vi "GetCellTypesAndValues.vi"(11 "XML":string) -> (2 "Type":string[](array[string]), 3 "Value":string[](array[string]))   [LabVIEW 2013]
uses:
  XML.lvlib
  <vilib>/xml/NI_XML.lvlib
  <resource>/objmgr/DOMUserDefRef.rc
panel:
  # "Output"
  # "Input"
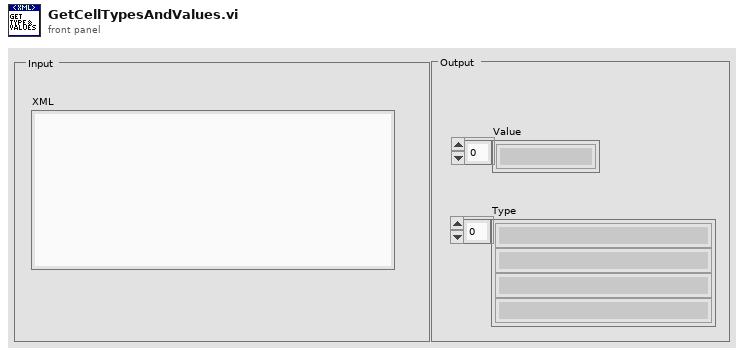
[diagram p1: front panel]
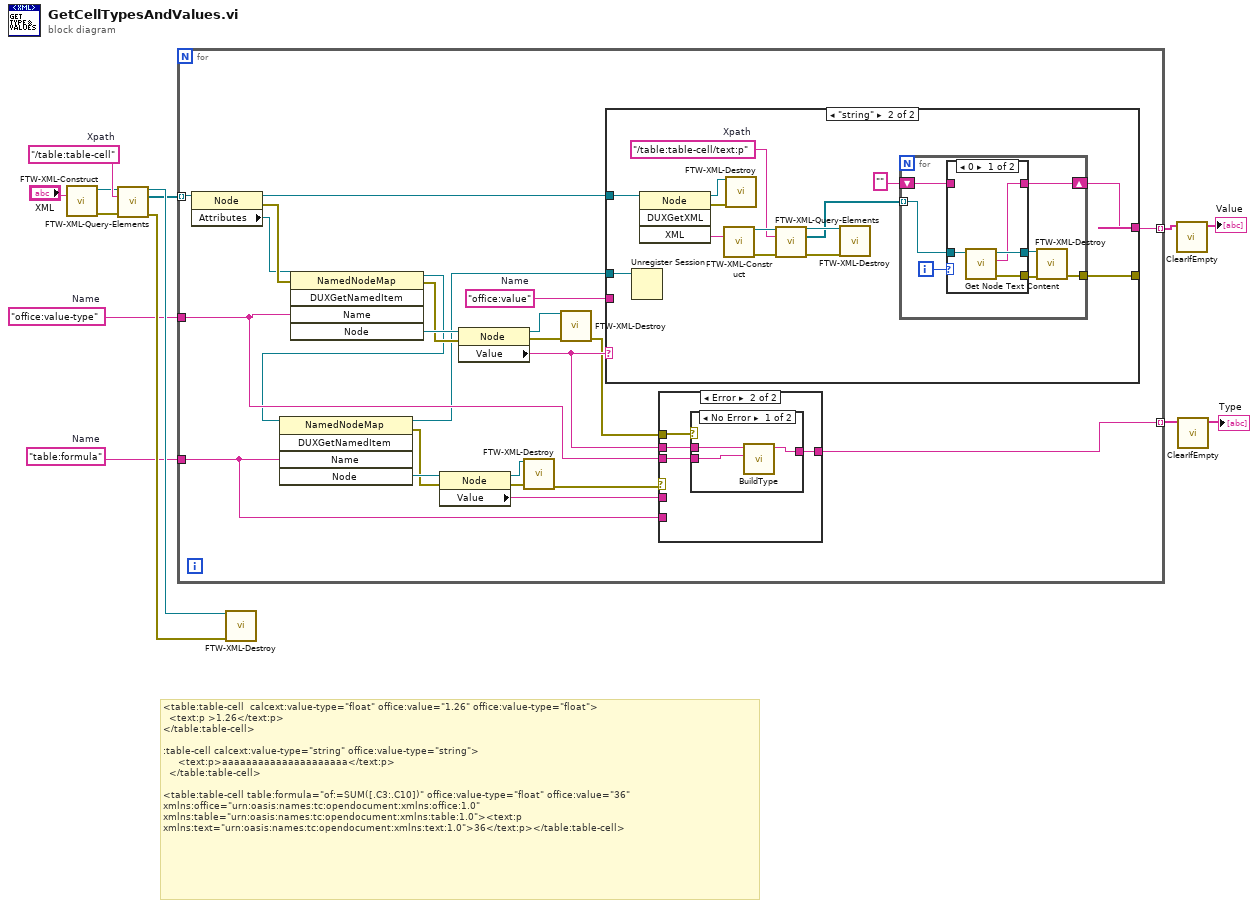
[diagram p0: block diagram]
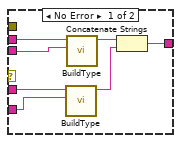
[diagram p2: hidden frame]
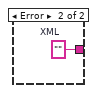
[diagram p3: hidden frame]
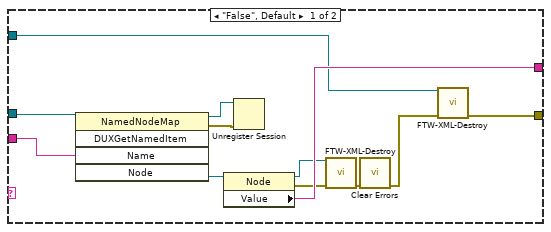
[diagram p4: hidden frame]
diagram:
  w5 = "table:formula"  # Name
  w6 = "office:value-type"  # Name
  w10 = "/table:table-cell"  # Xpath
  # "<table:table-cell  calcext:value-type=\"float\" office:value=\"1.26\" office:value-type=\"float\">\n  <text:p >1.26</text:p>\n</table:table-cell>\n\n:table-cell calcext:value-type=\"string\" office:value-type=\"string\">           \n     <text:p>aaaaaaaaaaaaaaaaaaaaa</text:p>\n  </table:table-cell>\n\n<table:table-cell table:formula=\"of:=SUM([.C3:.C10])\" office:value-type=\"float\" office:value=\"36\" xmlns:office=\"urn:oasis:names:tc:opendocument:xmlns:office:1.0\" xmlns:table=\"urn:oasis:names:tc:opendocument:xmlns:table:1.0\"><text:p xmlns:text=\"urn:oasis:names:tc:opendocument:xmlns:text:1.0\">36</text:p></table:table-cell>"
  n1 = call "FTW-XML-Construct.vi"("XML String"="XML") -> ("XML Document"=w8:refnum<k20>, "error out"=w9:errorcluster)  [unwired: 13 in]
  n2 = call "FTW-XML-Query-Elements.vi"("XML Node"=w8, "XPath Query"=w10, "error in"=w9) -> ("XML Node out"=w13:refnum<k20>, "Matching Nodes"=w11:refnum<k20>[], "error out"=w12:errorcluster)  [unwired: 9 in, 1 out]
  n3 = for {
    tunnel: [w36] -> w4 mode=indexing
    tunnel: w11 -> [w35] mode=indexing
    tunnel: w6 -> [w20]
    tunnel: [w23] -> w2 mode=indexing
    tunnel: w5 -> [w21]
    w29 = "office:value"  # Name
    n4 = property class="Node"(reference=w35) -> (reference out=w28:refnum<k20>, error out=w34:errorcluster, "Attributes"=w27:refnum<k20>)  [unwired: 1 in]
    n5 = invoke class="NamedNodeMap" method="DUXGetNamedItem"(reference=w27, error in=w34, "Name"=w20) -> (reference out=w15:refnum<k20>, error out=w30:errorcluster, "Node"=w33:refnum<k20>)  [unwired: 2 in, 2 out]
    n6 = invoke class="NamedNodeMap" method="DUXGetNamedItem"(reference=w15, "Name"=w21) -> (reference out=w14:refnum<k20>, error out=w25:errorcluster, "Node"=w26:refnum<k20>)  [unwired: 3 in, 2 out]
    n7 = property class="Node"(reference=w26, error in=w25) -> (reference out=w16:refnum<k20>, error out=w18:errorcluster, "Value"=w22:string)
    n8 = property class="Node"(reference=w33, error in=w30) -> (reference out=w31:refnum<k20>, error out=w32:errorcluster, "Value"=w24:string)
    n9 = call "FTW-XML-Destroy.vi"("XML Node"=w16, "error in"=w18) -> ("error out"=w17:errorcluster)  [unwired: 13 in]
    n10 = call "FTW-XML-Destroy.vi"("XML Node"=w31, "error in"=w32) -> ("error out"=w19:errorcluster)  [unwired: 13 in]
    n11 = case shown="\"string\"" w24 {
      tunnel: [w60 w65] -> w36
      tunnel: [w56 w77] -> _
      tunnel: w28 -> [w54 w76]
      tunnel: w14 -> [w63 w64]
      tunnel: w29 -> [w62 _]
      frame "False", Default {
        n12 = invoke class="NamedNodeMap" method="DUXGetNamedItem"(reference=w63, "Name"=w62) -> (reference out=w52:refnum<k20>, error out=w53:errorcluster, "Node"=w61:refnum<k20>)  [unwired: 3 in, 2 out]
        n13 = property class="Node"(reference=w61) -> (reference out=w58:refnum<k20>, error out=w59:errorcluster, "Value"=w60:string)  [unwired: 1 in]
        n14 = Unregister Session(8:w53, 11:w52) -> ()  [unwired: 1 out]
        n15 = call "FTW-XML-Destroy.vi"("XML Node"=w58, "error in"=w59) -> ("error out"=w57:errorcluster)  [unwired: 13 in]
        n16 = call <vilib>:"Clear Errors.vi"("error in (no error)"=w57) -> ("error out"=w55:errorcluster)  [unwired: 6 in]
        n17 = call "FTW-XML-Destroy.vi"("XML Node"=w54, "error in"=w55) -> ("error out"=w56:errorcluster)  [unwired: 13 in]
      }
      frame "string" {
        w69 = "/table:table-cell/text:p"  # Xpath
        n18 = Unregister Session(11:w64) -> ()  [unwired: 1 in, 1 out]
        n19 = invoke class="Node" method="DUXGetXML"(reference=w76) -> (reference out=w67:refnum<k20>, error out=w68:errorcluster, "XML"=w75:string)  [unwired: 3 in, 1 out]
        n20 = call "FTW-XML-Construct.vi"("XML String"=w75) -> ("XML Document"=w74:refnum<k20>, "error out"=w73:errorcluster)  [unwired: 13 in]
        n21 = call "FTW-XML-Destroy.vi"("XML Node"=w67, "error in"=w68) -> ()  [unwired: 13 in, 1 out]
        n22 = call "FTW-XML-Query-Elements.vi"("XML Node"=w74, "XPath Query"=w69, "error in"=w73) -> ("XML Node out"=w71:refnum<k20>, "Matching Nodes"=w70:refnum<k20>[], "error out"=w72:errorcluster)  [unwired: 9 in, 1 out]
        n23 = call "FTW-XML-Destroy.vi"("XML Node"=w71, "error in"=w72) -> ()  [unwired: 13 in, 1 out]
        n24 = for {
          tunnel: [w80] -> w77
          tunnel: w70 -> [w84] mode=indexing
          shift-right: [w81] -> w65
          shift-left: "" -> [w83]
          i -> [w82]
          n25 = case shown="0" w82 {
            tunnel: [w88 _] -> w79
            tunnel: w84 -> [w87 w89]
            tunnel: [w86 w89] -> w78
            tunnel: w83 -> [_ w90]
            tunnel: [w85 w90] -> w81
            frame 0 {
              n26 = call <vilib>:"Get Node Text Content.vi"("node in"=w87) -> ("error out"=w88:errorcluster, "node text"=w85:string, "node out"=w86:refnum<k20>)  [unwired: 8 in]
            }
            frame 1, Default {
            }
          }
          n27 = call "FTW-XML-Destroy.vi"("XML Node"=w78, "error in"=w79) -> ("error out"=w80:errorcluster)  [unwired: 13 in]
        }
      }
    }
    n28 = case shown="Error" w17 {
      tunnel: w24 -> [w39 w46]
      tunnel: [w41 w45] -> w23
      tunnel: w22 -> [w38 _]
      tunnel: w21 -> [w37 _]
      tunnel: w20 -> [w40 w47]
      tunnel: w19 -> [_ w44]
      frame No Error {
        n29 = call "BuildType.vi"("Tag"=w37, "Value"=w38) -> ("XML"=w42:string)  [unwired: 9 in]
        n30 = call "BuildType.vi"("Tag"=w40, "Value"=w39) -> ("XML"=w43:string)  [unwired: 9 in]
        n31 = Concatenate Strings(w43, w42) -> (w41:string)
      }
      frame Error {
        n32 = case shown="No Error" w44 {
          tunnel: w47 -> [w50 _]
          tunnel: w46 -> [w49 _]
          tunnel: [w48 w51] -> w45
          frame No Error {
            n33 = call "BuildType.vi"("Tag"=w50, "Value"=w49) -> ("XML"=w48:string)  [unwired: 9 in]
          }
          frame Error {
            w51 = ""  # XML
          }
        }
      }
    }
  }
  n34 = call "FTW-XML-Destroy.vi"("XML Node"=w13, "error in"=w12) -> ()  [unwired: 13 in, 1 out]
  n35 = call "ClearIfEmpty.vi"("Array"=w4) -> ("ArrayOut"=→"Value":string[])  [unwired: 10 in]
  n36 = call "ClearIfEmpty.vi"("Array"=w2) -> ("ArrayOut"=→"Type":string[])  [unwired: 10 in]
